vi "binary.vi"() -> ()   [LabVIEW 2020]
uses:
  <vilib>/Utility/error.llb/DialogType.ctl
panel:
  out "data":dbl[](array[numeric])
  out "Array":dbl[](array[numeric])
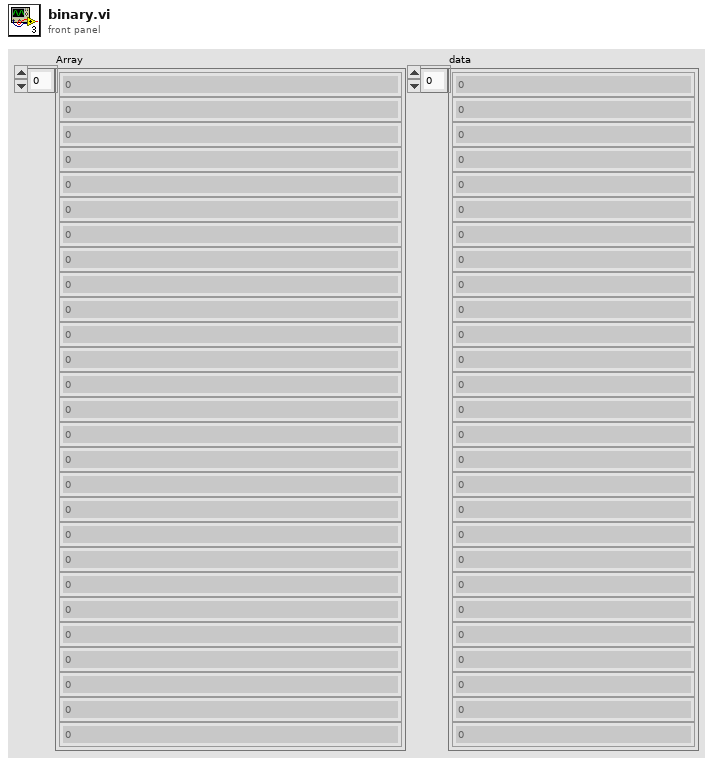
[diagram p1: front panel]
types:
  T1 = enum16{"open", "replace", "create", "open or create", "replace or create", "replace or create with confirmation"}
  T2 = typedef "DialogType.ctl" = u16
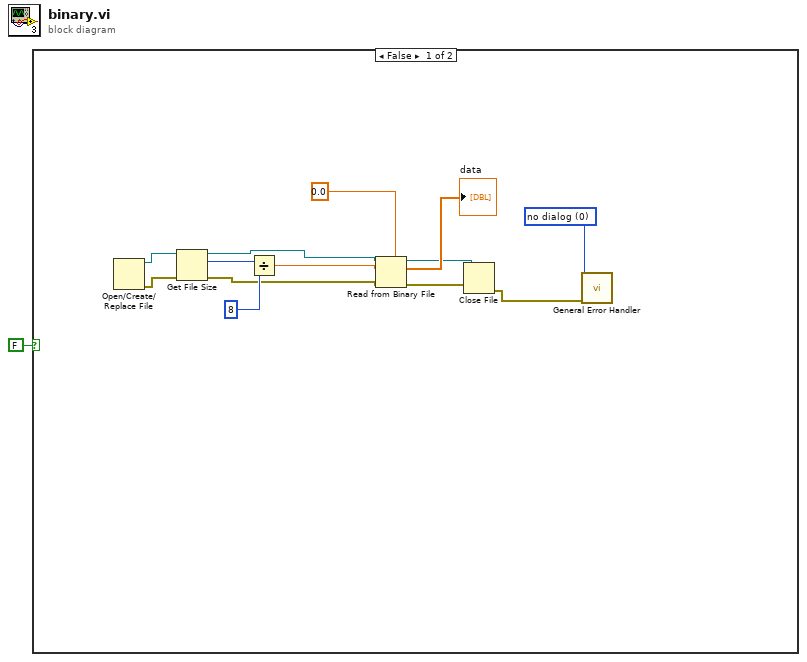
[diagram p0: block diagram]
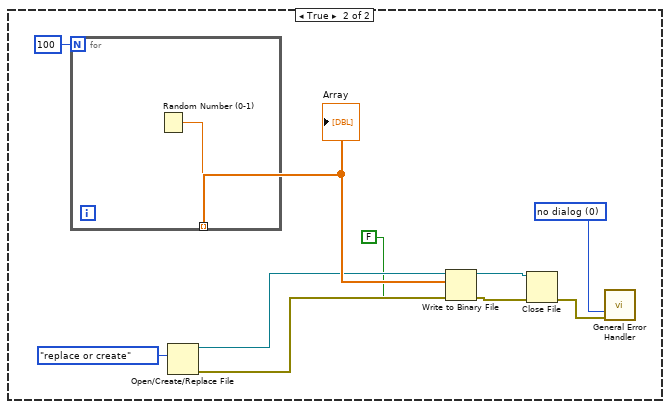
[diagram p2: hidden frame]
diagram:
  n1 = case shown="False" FALSE {
    frame False {
      w2 = T2 0 items=["no dialog", "OK message", "continue or stop message", "OK message + warnings", "continue/stop + warnings"] ("type of dialog (OK msg:1)")
      n2 = Open/Create/Replace File() -> (refnum out=w13:refnum<file>, error out=w14:errorcluster)  [unwired: 6 in, 1 out]
      n3 = Get File Size(file=w13, error in=w14) -> (refnum out=w10:refnum<file>, size (in bytes)=w12:i64, 0:w8:errorcluster)
      n4 = Divide(x=w12, y=i64 8) -> (x/y=w9:dbl)
      n5 = Read from Binary File(5:0.0, 8:w8, 10:w9, 11:w10) -> (0:w5:errorcluster, 2:→"data":dbl[], 3:w4:refnum<file>)  [unwired: 2 in, 1 out]
      n6 = Close File(refnum=w4, error in=w5) -> (error out=w3:errorcluster)  [unwired: 1 out]
      n7 = call <vilib>:"General Error Handler.vi"("type of dialog (OK msg:1)"=w2, "error in (no error)"=w3) -> ()  [unwired: 9 in, 5 out]
    }
    frame True {
      w15 = T2 0 items=["no dialog", "OK message", "continue or stop message", "OK message + warnings", "continue/stop + warnings"] ("type of dialog (OK msg:1)")
      n8 = for {
        N: 100 -> [_]
        tunnel: [w25] -> w22 mode=indexing
        n9 = Random Number (0-1)() -> (number: 0 to 1=w25:dbl)
      }
      "Array" <- w22
      n10 = Open/Create/Replace File(operation (0:open)=T1."replace or create") -> (refnum out=w21:refnum<file>, error out=w20:errorcluster)  [unwired: 5 in, 1 out]
      n11 = Write to Binary File(file (use dialog)=w21, data=w22, error in=w20, 5:FALSE) -> (refnum out=w17:refnum<file>, error out=w18:errorcluster)  [unwired: 2 in, 1 out]
      n12 = Close File(refnum=w17, error in=w18) -> (error out=w16:errorcluster)  [unwired: 1 out]
      n13 = call <vilib>:"General Error Handler.vi"("type of dialog (OK msg:1)"=w15, "error in (no error)"=w16) -> ()  [unwired: 9 in, 5 out]
    }
  }
